vi "Read heating control.vi"(8 "error in (no error)":errorcluster, 10 "value":string, 11 "HT_in in":T1 {"Y_H" step=1.0; "SP" step=0.01 format="%.2f"}) -> (0 "error out":errorcluster, 2 "Data to Write":bool, 3 "HT1_in out":T1 {"Y_H" step=1.0; "SP" step=0.01 format="%.2f"})   [LabVIEW 2019, in "Heating.lvlib"]
uses:
  Heating.lvlib
  ctl/ZY_control.ctl
  Reg/ctl/Z_State.ctl
  Reg/ctl/Y_state.ctl
  ctl/Z_State.ctl
  ctl/Y_state.ctl
  <vilib>/JDP Science/JSONtext/String Subset.vi
  <vilib>/JDP Science/JSONtext/support/Strip Quotes and Unescape.vi
  <vilib>/JDP Science/JSONtext/Parsing/Parse Full Path or Item Name.vi
  <vilib>/JDP Science/JSONtext/Offset/Find Item Locations by Path.vi
  <vilib>/JDP Science/JSONtext/support/Unescape JSON string.vi
  <vilib>/JDP Science/JSONtext/JSONtext.lvlib
  Reg/control.lvlib
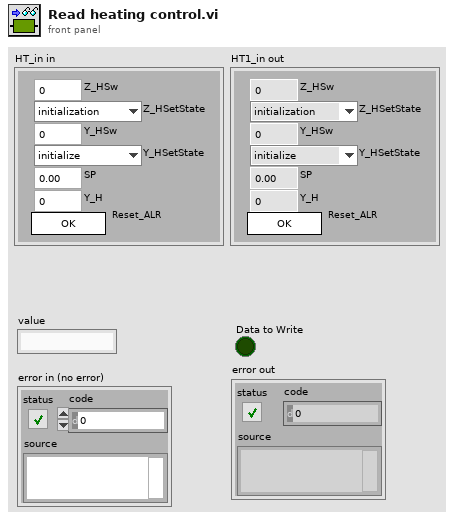
[diagram p1: front panel]
types:
  T1 = typedef "Heating.lvlib/ZY_control.ctl" = cluster{"Z_HSw":u32, "Z_HSetState":T2, "Y_HSw":u32, "Y_HSetState":T3, "SP":dbl, "Y_H":dbl, "Reset_ALR":bool}
  T2 = typedef "control.lvlib/Z_State.ctl" = enum8{"initialization", "alarm", "disabled", "not ready", "stop ready", "reserv", "switched off", "reserv2", "switched on", "check", "on min", "decrease out", "on", "increase out", "on max"}
  T3 = typedef "control.lvlib/Y_state.ctl" = enum8{"initialize", "alarm", "min", "stop", "hand", "auto", "max"}
  T4 = typedef "Heating.lvlib/Z_State.ctl" = enum8{"initialization", "alarm", "disabled", "not ready", "stop ready", "reserv", "switched off", "reserv2", "switched on", "check", "on min", "decrease out", "on", "increase out", "on max"}
  T5 = typedef "Heating.lvlib/Y_state.ctl" = enum8{"initialize", "alarm", "min", "stop", "hand", "auto", "max"}
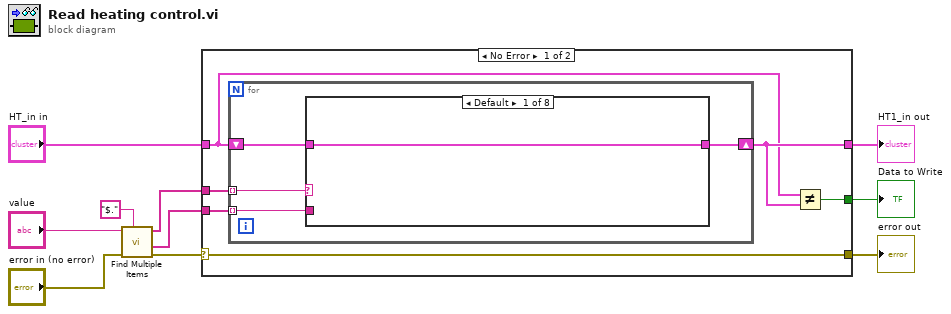
[diagram p0: block diagram]
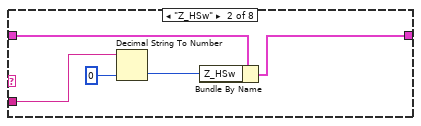
[diagram p2: hidden frame]
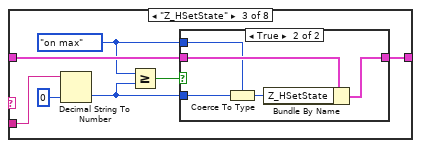
[diagram p3: hidden frame]
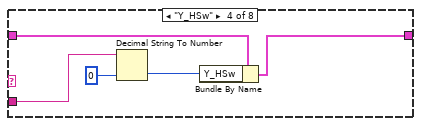
[diagram p5: hidden frame]
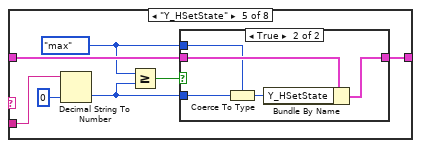
[diagram p6: hidden frame]
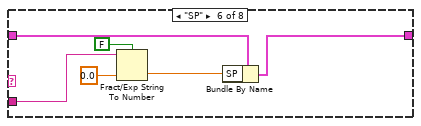
[diagram p8: hidden frame]
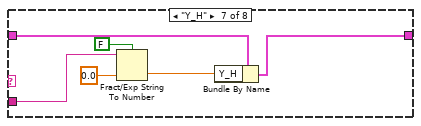
[diagram p9: hidden frame]
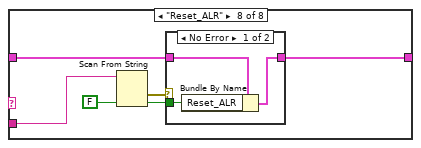
[diagram p10: hidden frame]
diagram:
  n1 = call <vilib>:"Find Multiple Items.vi"("$Path or Item Name"="$.", "error in (no error)"="error in (no error)", "JSON"="value") -> ("error out"=w7:errorcluster, "<JSON>"=w5:string[], "Item Names"=w10:string[])  [unwired: 5 in, 1 out]
  n2 = case shown="No Error" w7 {
    selector: w7 -> [w13 w80]
    tunnel: w10 -> [w16 _]
    tunnel: "HT_in in" -> [w11 w81]
    tunnel: w5 -> [w15 _]
    tunnel: [w12 w81] -> w6
    tunnel: [w14 _] -> w2
    tunnel: [w13 w80] -> w1
    frame No Error {
      n3 = for {
        shift-right: [w18] -> w12
        shift-left: w11 -> [w20]
        tunnel: w16 -> [w17] mode=indexing
        tunnel: w15 -> [w19] mode=indexing
        n4 = case shown="Default" w17 {
          tunnel: w20 -> [w21 w26 w33 w44 w51 w63 w69 w75]
          tunnel: w19 -> [_ w23 w31 w41 w49 w60 w66 w72]
          tunnel: [w21 w22 w30 w40 w48 w59 w65 w74] -> w18
          frame Default {
          }
          frame "Z_HSw" {
            n5 = Decimal String To Number(string=w23, default (0L)=u32 0 ("Z_HSw")) -> (number=w24:u32)  [unwired: 1 in, 1 out]
            n6 = Bundle By Name(cluster=w26, "Z_HSw"=w24) -> (w22:T1)
          }
          frame "Z_HSetState" {
            w29 = Z_State."on max" ("Z_HSetState")
            n7 = Decimal String To Number(string=w31, default (0L)=u8 0 ("Z_HSw")) -> (number=w27:u8)  [unwired: 1 in, 1 out]
            n8 = Greater Or Equal?(x=w29, y=w27) -> (x >= y?=w28:bool)
            n9 = case shown="True" w28 {
              tunnel: w33 -> [w34 w39]
              tunnel: [w34 w38] -> w30
              tunnel: w29 -> [_ w36]
              tunnel: w27 -> [_ w35]
              frame False {
              }
              frame True {
                n10 = Coerce To Type(0:w35, 1:w36) -> (2:w37:T4)
                n11 = Bundle By Name(cluster=w39, "Z_HSetState"=w37) -> (w38:T1)
              }
            }
          }
          frame "Y_HSw" {
            n12 = Decimal String To Number(string=w41, default (0L)=u32 0 ("Z_HSw")) -> (number=w42:u32)  [unwired: 1 in, 1 out]
            n13 = Bundle By Name(cluster=w44, "Y_HSw"=w42) -> (w40:T1)
          }
          frame "Y_HSetState" {
            w45 = Y_state."max" ("Y_HSetState")
            n14 = Decimal String To Number(string=w49, default (0L)=u8 0 ("Z_HSw")) -> (number=w46:u8)  [unwired: 1 in, 1 out]
            n15 = Greater Or Equal?(x=w45, y=w46) -> (x >= y?=w47:bool)
            n16 = case shown="True" w47 {
              tunnel: w51 -> [w52 w57]
              tunnel: [w52 w56] -> w48
              tunnel: w45 -> [_ w54]
              tunnel: w46 -> [_ w53]
              frame False {
              }
              frame True {
                n17 = Coerce To Type(0:w53, 1:w54) -> (2:w55:T5)
                n18 = Bundle By Name(cluster=w57, "Y_HSetState"=w55) -> (w56:T1)
              }
            }
          }
          frame "SP" {
            n19 = Fract/Exp String To Number(use system decimal point (T)=FALSE, string=w60, default (0 dbl)=0.0 ("Z_HSw")) -> (number=w61:dbl)  [unwired: 1 in, 1 out]
            n20 = Bundle By Name(cluster=w63, "SP"=w61) -> (w59:T1)
          }
          frame "Y_H" {
            n21 = Fract/Exp String To Number(use system decimal point (T)=FALSE, string=w66, default (0 dbl)=0.0 ("Z_HSw")) -> (number=w67:dbl)  [unwired: 1 in, 1 out]
            n22 = Bundle By Name(cluster=w69, "Y_H"=w67) -> (w65:T1)
          }
          frame "Reset_ALR" {
            n23 = Scan From String(input string=w72, default 1=FALSE ("use system decimal point (T)")) -> (error out=w70:errorcluster, output 1=w71:bool)  [unwired: 3 in, 2 out]
            n24 = case shown="No Error" w70 {
              tunnel: w75 -> [w78 w79]
              tunnel: [w77 w79] -> w74
              tunnel: w71 -> [w76 _]
              frame No Error {
                n25 = Bundle By Name(cluster=w78, "Reset_ALR"=w76) -> (w77:T1)
              }
              frame Error {
              }
            }
          }
        }
      }
      n26 = Not Equal?(x=w11, y=w12) -> (x != y?=w14:bool)
    }
    frame Error {
    }
  }
  "HT1_in out" <- w6
  "Data to Write" <- w2
  "error out" <- w1
